vi "ChangeComboCellValues.vi"(10 "index":i32, 11 "ColumnSetup in":T1[](array[typedef]) {"MinWidth" min=2 step=1; "AutoSizeMode" items=["None"=1, "ColumnHeader"=2, "AllCellsExceptHeader"=4, "AllCells"=6, "DisplayedCellsExceptHeader"=8, "DisplayedCells"=10, "Fill"=16]; "FillWeight" min=1 max=100}) -> (3 "ColumnSetup out":T1[](array[typedef]) {"MinWidth" min=2 step=1; "AutoSizeMode" items=["None"=1, "ColumnHeader"=2, "AllCellsExceptHeader"=4, "AllCells"=6, "DisplayedCellsExceptHeader"=8, "DisplayedCells"=10, "Fill"=16]; "FillWeight" min=1 max=100})   [LabVIEW 2013]
uses:
  Shared/LabVIEWdotNetDataGrid-master/source/GridColumn/ColumnDefinition.ctl
  Shared/LabVIEWdotNetDataGrid-master/source/GridColumn/ColumnType.ctl
  Shared/LabVIEWdotNetDataGrid-master/source/GridColumn/GridColumn.lvclass
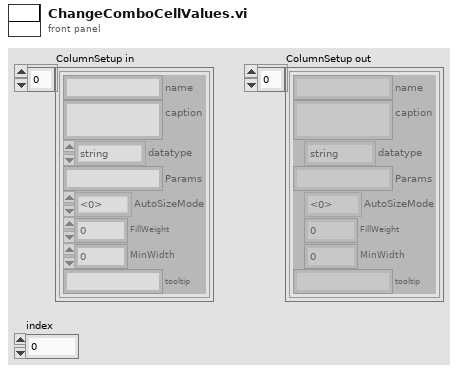
[diagram p1: front panel]
types:
  T1 = typedef "DataGrid.lvlib/GridColumn.lvclass/ColumnDefinition.ctl" = cluster{"name":string, "caption":string, "datatype":T2, "Params":string, "AutoSizeMode":i32, "FillWeight":sgl, "MinWidth":u32, "tooltip":string}
  T2 = typedef "DataGrid.lvlib/GridColumn.lvclass/ColumnType.ctl" = enum16{"string", "image", "check", "numeric", "timestamp", "button", "combo", "link"}
  T3 = typedef "mysql_authentication.ctl" = cluster{"User":string, "Password":string, "Database":string}
  T4 = cluster{"Port":u16, "IP Address":string, "Authentication":T3}
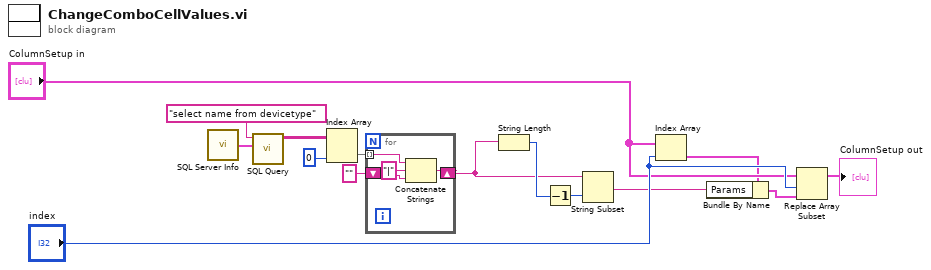
[diagram p0: block diagram]
diagram:
  n1 = call "SQL Server Info.vi"() -> ("SQL Server Info"=w4:T4)
  n2 = call "SQL Query.vi"("SQL Server Info"=w4, "Query"="select name from devicetype") -> ("data"=w2:string[][])  [unwired: 8 in, 1 out]
  n3 = Index Array(array=w2, index (col)=0 ("disabled index (col)")) -> (element=w5:string[])  [unwired: 1 in]
  n4 = for {
    tunnel: w5 -> [w19] mode=indexing
    shift-right: [w17] -> w8
    shift-left: "" -> [w16]
    n5 = Concatenate Strings(w19, "|" ("string"), w16) -> (w17:string)
  }
  n6 = String Length(string=w8) -> (length=w9:i32)
  n7 = Decrement(x=w9) -> (x-1=w7:i32)
  n8 = String Subset(string=w8, length (rest)=w7) -> (substring=w11:string)  [unwired: 1 in]
  n9 = Index Array(array="ColumnSetup in", index="index") -> (element=w10:T1)
  n10 = Bundle By Name(cluster=w10, "Params"=w11) -> (w13:T1)
  n11 = Replace Array Subset(array="ColumnSetup in", new element=w13, index="index") -> (→"ColumnSetup out":T1[])
